vi "Set Rendezvous ref.vi"(8 "error in (no error)":errorcluster, 10 "rendezvous":T1, 11 "Philosopher in":refnum<class "Philosopher.lvclass">) -> (0 "error out":errorcluster, 3 "Philosopher out":refnum<class "Philosopher.lvclass">)   [LabVIEW 2023, in "Philosopher.lvlib" / "Philosopher.lvclass"]
uses:
  Philosopher.lvclass
  Philosopher.lvclass/Philosopher.ctl
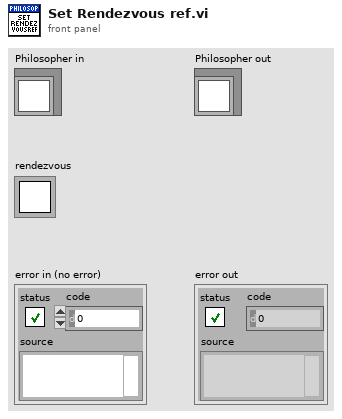
[diagram p1: front panel]
types:
  T1 = typedef "Rendezvous RefNum" = refnum<k1>
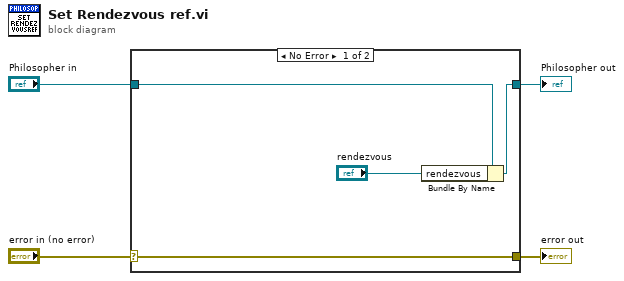
[diagram p0: block diagram]
diagram:
  n1 = case shown="No Error" "error in (no error)" {
    selector: "error in (no error)" -> [w8 w9]
    tunnel: [w8 w9] -> w3
    tunnel: [w6 w10] -> w1
    tunnel: "Philosopher in" -> [w7 w10]
    frame No Error {
      n2 = Bundle By Name(cluster=w7, "rendezvous"="rendezvous") -> (w6:refnum<class "Philosopher.lvclass">)
    }
    frame Error {
    }
  }
  "error out" <- w3
  "Philosopher out" <- w1
